vi "ReadTuidCertid.vi"(8 "error in":errorcluster caption="错误输入", 9 "ICCID":string="1805", 10 "SN":string="1805", 11 "PartN":string="1805") -> (0 "error out":errorcluster caption="错误输出", 1 "Certid":string, 2 "TUID":string, 3 "ReportStrA":string)   [LabVIEW 2013]
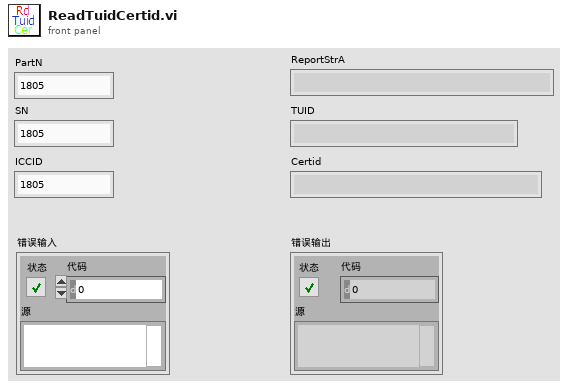
[diagram p1: front panel]
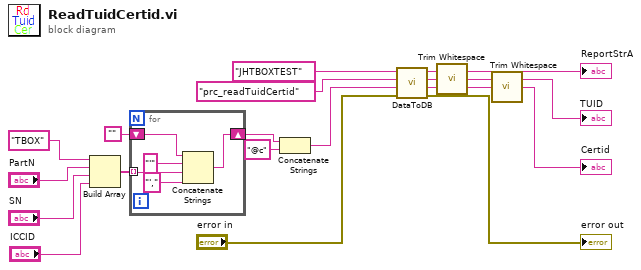
[diagram p0: block diagram]
diagram:
  n1 = Build Array("TBOX" ("DeviceType"), "PartN", "SN", "ICCID") -> (w15:string[])
  n2 = for {
    shift-right: [w22] -> w14
    shift-left: "" -> [w23]
    tunnel: w15 -> [w19] mode=indexing
    n3 = Concatenate Strings(w23, "'", w19, "',") -> (w22:string)
  }
  n4 = Concatenate Strings(w14, "@c" ("字符串")) -> (w10:string)
  n5 = call "DataToDB.vi"("error in"="error in", "all string"=w10, "Procedure name"="prc_readTuidCertid", "DSN name"="JHTBOXTEST") -> ("error out"=→"error out":errorcluster, "Certid"=w5:string, "TUID"=w6:string, "ReportStrA"=→"ReportStrA":string)  [unwired: 4 in]
  n6 = call <vilib>:"Trim Whitespace.vi"("string"=w6) -> ("trimmed string"=→"TUID":string)  [unwired: 1 in]
  n7 = call <vilib>:"Trim Whitespace.vi"("string"=w5) -> ("trimmed string"=→"Certid":string)  [unwired: 1 in]
